vi "RightClickUpdate.vi"(8 "error in (no error)":errorcluster, 10 "Refs":T12, 11 "Loop data in":T1={"TitleCollapse"=refnum, "MouseDownState"=enum."Idle", "RightClickCache"={"Mod"={"Ctrl"=FALSE, "Shift"=FALSE}, "CoordsStart"={"Horizontal"=0, "Vertical"=0}, "CoordsEnd"={"Horizontal"=0, "Vertical"=0}, "PlotAreaBounds"={"Left"=10, "Top"=10, "Right"=0, "Bottom"=0}, "slice"=[]}, "ZoomCache"={"SuppressedPlots"=[], "LeftAxis"={"NeedsRevert?"=FALSE, "Scale Fit"=0, "Range"={"Minimum"=0.0, "Maximum"=0.0, "Increment"=0.0, "Minor Increment"=0.0, "Start"=0.0}}, "RightAxis"={"NeedsRevert?"=FALSE, "Scale Fit"=0, "Range"={"Minimum"=0.0, "Maximum"=0.0, "Increment"=0.0, "Minor Increment"=0.0, "Start"=0.0}}, "Mod"={"Shift"=FALSE}}, "UpdateTime"=0.0, "keyboard"=refnum, "visible?"=FALSE}) -> (0 "error out":errorcluster, 3 "Loop data out":T1={"TitleCollapse"=refnum, "MouseDownState"=enum."Idle", "RightClickCache"={"Mod"={"Ctrl"=FALSE, "Shift"=FALSE}, "CoordsStart"={"Horizontal"=0, "Vertical"=0}, "CoordsEnd"={"Horizontal"=0, "Vertical"=0}, "PlotAreaBounds"={"Left"=10, "Top"=10, "Right"=0, "Bottom"=0}, "slice"=[]}, "ZoomCache"={"SuppressedPlots"=[], "LeftAxis"={"NeedsRevert?"=FALSE, "Scale Fit"=0, "Range"={"Minimum"=0.0, "Maximum"=0.0, "Increment"=0.0, "Minor Increment"=0.0, "Start"=0.0}}, "RightAxis"={"NeedsRevert?"=FALSE, "Scale Fit"=0, "Range"={"Minimum"=0.0, "Maximum"=0.0, "Increment"=0.0, "Minor Increment"=0.0, "Start"=0.0}}, "Mod"={"Shift"=FALSE}}, "UpdateTime"=0.0, "keyboard"=refnum, "visible?"=FALSE})   [LabVIEW 2021, in "RocketPlot.lvlib"]
uses:
  RocketPlot.lvlib
  TypeDefs/Plot UI references.ctl
  Classes/RocketPlotHandle/RocketPlotHandle.lvclass
  <userlib>/bjustice/TipStripOOPanel/Classes/TipPanelHandle/TipPanelHandle.lvclass
  TypeDefs/Plot top row.ctl
  TypeDefs/plot while loop data.ctl
  CollapsePanel/CollapsePanel.lvclass
  TypeDefs/MouseDownState.ctl
  TypeDefs/RightClickCache.ctl
  TypeDefs/RightClickCache PlatMod.ctl
  <vilib>/Utility/miscctls.llb/LVPoint32TypeDef.ctl
  <vilib>/Utility/miscctls.llb/LVRectTypeDef.ctl
  TypeDefs/Slice average.ctl
  TypeDefs/ZoomCache.ctl
  TypeDefs/RangeCache.ctl
  <vilib>/Utility/miscctls.llb/LVRangeTypeDef.ctl
  TypeDefs/ZoomCache PlatMod.ctl
  Plot Load maker V2 - scaleread grid colors.vi
  Classes/TipTablePanel/new cell.vi
  Plot scale refnum to LUT name.vi
  Classes/TipTablePanel/TipTablePanel.lvclass
  C:/Program Files/National Instruments/LabVIEW 2021/user.lib/bjustice/TipStripOOPanel/Classes/TipPanel/TipPanel.lvclass
  <userlib>/bjustice/TipStripOOPanel/Classes/TipPanelHandle/CMD - hide.vi
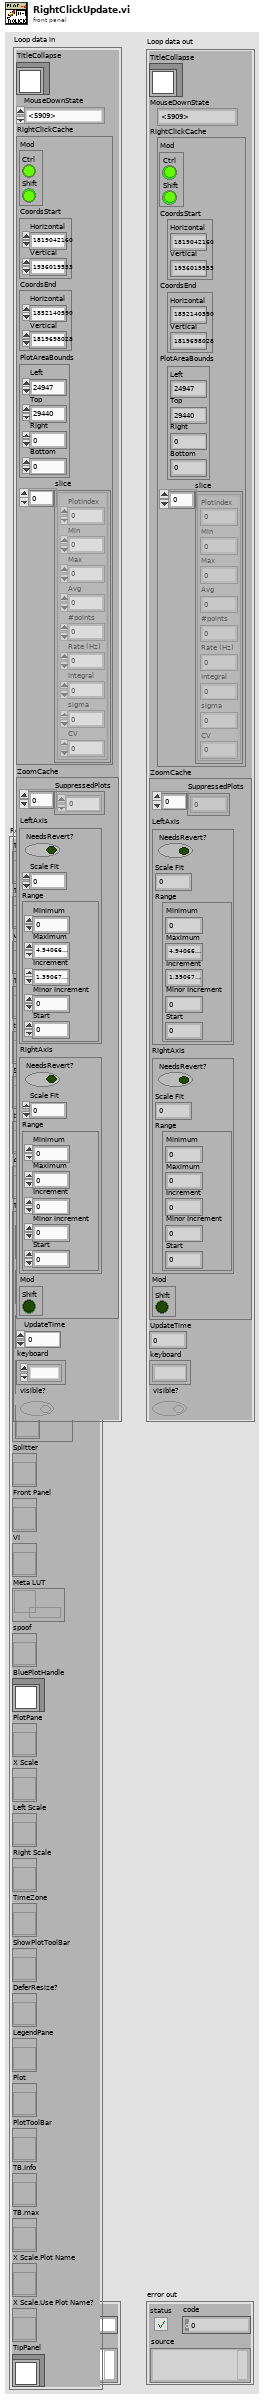
[diagram p1: front panel]
types:
  T1 = typedef "RocketPlot.lvlib/plot while loop data.ctl" = cluster{"TitleCollapse":refnum<class "CollapsePanel.lvclass">, "MouseDownState":T2, "RightClickCache":T3, "ZoomCache":T8, "UpdateTime":dbl, "keyboard":refnum<k1>, "visible?":bool}
  T2 = typedef "RocketPlot.lvlib/MouseDownState.ctl" = enum16{"Idle", "Pan", "Zoom", "Zoom-Post", "RightClick"}
  T3 = typedef "RocketPlot.lvlib/RightClickCache.ctl" = cluster{"Mod":T4, "CoordsStart":T5, "CoordsEnd":T5, "PlotAreaBounds":T6, "slice":T7[]}
  T4 = typedef "RocketPlot.lvlib/RightClickCache PlatMod.ctl" = cluster{"Ctrl":bool, "Shift":bool}
  T5 = typedef "LVPoint32TypeDef.ctl" = cluster{"Horizontal":i32, "Vertical":i32}
  T6 = typedef "LVRectTypeDef.ctl" = cluster{"Left":i16, "Top":i16, "Right":i16, "Bottom":i16}
  T7 = typedef "RocketPlot.lvlib/Slice average.ctl" = cluster{"PlotIndex":i32, "Min":dbl, "Max":dbl, "Avg":dbl, "#points":u32, "Rate (Hz)":dbl, "Integral":dbl, "sigma":dbl, "CV":dbl}
  T8 = typedef "RocketPlot.lvlib/ZoomCache.ctl" = cluster{"SuppressedPlots":i32[], "LeftAxis":T9, "RightAxis":T9, "Mod":T11}
  T9 = typedef "RocketPlot.lvlib/RangeCache.ctl" = cluster{"NeedsRevert?":bool, "Scale Fit":u8, "Range":T10}
  T10 = typedef "LVRangeTypeDef.ctl" = cluster{"Minimum":dbl, "Maximum":dbl, "Increment":dbl, "Minor Increment":dbl, "Start":dbl}
  T11 = typedef "RocketPlot.lvlib/ZoomCache PlatMod.ctl" = cluster{"Shift":bool}
  T12 = typedef "RocketPlot.lvlib/Plot UI references.ctl" = cluster{"Title":refnum<vi>, "Title?":refnum<vi>, "Visible sidebar?":refnum<vi>, "Time to Plot":refnum<vi>, "top array":refnum<vi>, "Scrollbar":refnum<vi>, "tab ref":refnum<vi>, "Add row":refnum<vi>, "TopArray":cluster{"PID":refnum<vi>, "Numeric color":refnum<vi>, "Flat":refnum<vi>, "PID color":refnum<vi>, "Data":refnum<vi>}, "Splitter":refnum<vi>, "Front Panel":refnum<vi>, "VI":refnum<vi>, "Meta LUT":refnum<data-value>, "spoof":refnum<vi>, "BluePlotHandle":refnum<class "RocketPlotHandle.lvclass">, "PlotPane":refnum<vi>, "X Scale":refnum<vi>, "Left Scale":refnum<vi>, "Right Scale":refnum<vi>, "TimeZone":refnum<vi>, "ShowPlotToolBar":refnum<vi>, "DeferResize?":refnum<vi>, "LegendPane":refnum<vi>, "Plot":refnum<vi>, "PlotToolBar":refnum<vi>, "TB.Info":refnum<vi>, "TB.max":refnum<vi>, "X Scale.Plot Name":refnum<vi>, "X Scale.Use Plot Name?":refnum<vi>, "TipPanel":refnum<class "TipPanelHandle.lvclass">}
  T13 = typedef "RocketPlot.lvlib/RightClickType.ctl" = enum16{"Idle", "Delta", "SliceAvg", "Identify"}
  T14 = typedef "RocketPlot.lvlib/TipTablePanel.lvclass/cell cache.ctl" = cluster{"text":string, "Color":u32, "Justification":enum16{"Left", "Center", "Right"}}
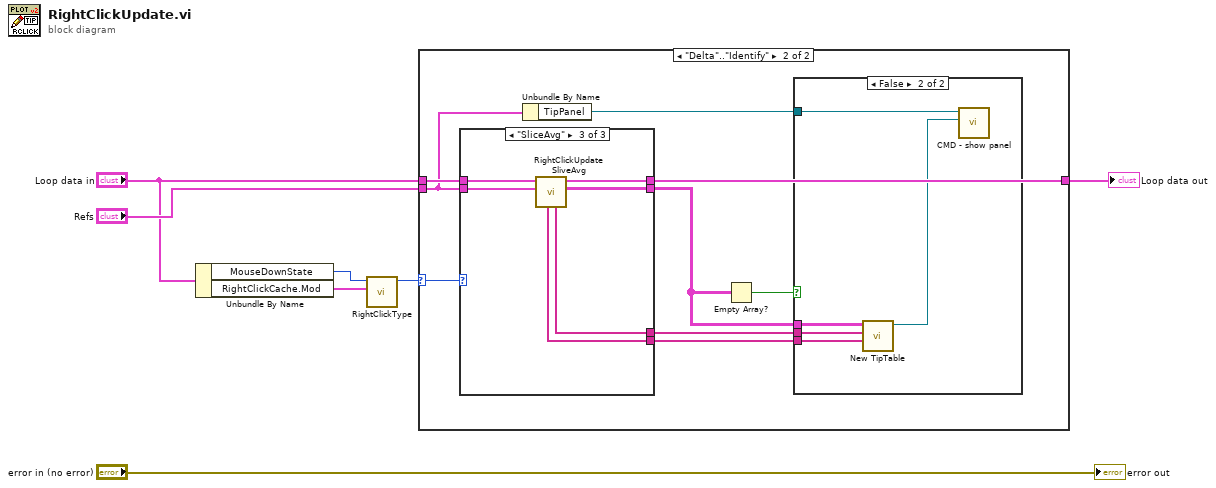
[diagram p0: block diagram]
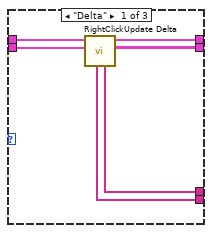
[diagram p3: hidden frame]
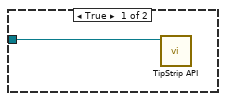
[diagram p5: hidden frame]
diagram:
  n1 = Unbundle By Name("Loop data in") -> ("MouseDownState"=w4:T2, "RightClickCache.Mod"=w5:T4)
  n2 = call "RightClickType.vi"("Mod"=w5, "MouseDownState"=w4) -> ("RightClickType"=w3:T13)  [unwired: 9 in]
  n3 = case shown="\"Delta\"..\"Identify\"" w3 {
    selector: w3 -> [_ w11]
    tunnel: "Refs" -> [_ w10]
    tunnel: "Loop data in" -> [w8 w16]
    tunnel: [w8 w12] -> w1
    frame "Idle" {
    }
    frame "Delta".."Identify" {
      n4 = case shown="\"SliceAvg\"" w11 {
        tunnel: w16 -> [w23 w24 w30]
        tunnel: w10 -> [w22 _ w28]
        tunnel: [w21 _ w27] -> w15
        tunnel: [w20 _ w25] -> w14
        tunnel: [w19 _ w26] -> w13
        tunnel: [w18 w24 w29] -> w12
        frame "Delta" {
          n5 = call "RightClickUpdate Delta.vi"("Refs"=w22, "Loop data in"=w23) -> ("cells"=w21:T14[][], "Loop data out"=w18:T1, "Row Headers"=w20:string[], "Column Headers"=w19:string[])  [unwired: 5 in, 1 out]
        }
        frame Default {
        }
        frame "SliceAvg" {
          n6 = call "RightClickUpdate SliveAvg.vi"("Refs"=w28, "Loop data in"=w30) -> ("cells"=w27:T14[][], "Loop data out"=w29:T1, "Row Headers"=w25:string[], "Column Headers"=w26:string[])  [unwired: 5 in, 1 out]
        }
      }
      n7 = Unbundle By Name(w10) -> ("TipPanel"=w9:refnum<class "TipPanelHandle.lvclass">)
      n8 = Empty Array?(array=w15) -> (empty?=w17:bool)
      n9 = case shown="False" w17 {
        tunnel: w14 -> [_ w35]
        tunnel: w13 -> [_ w34]
        tunnel: w15 -> [_ w36]
        tunnel: w9 -> [w31 w33]
        frame True {
          n10 = call-poly <userlib>:"TipStrip API.vi"("TipPanelHandle"=w31) -> ()  [unwired: 9 in, 2 out]
        }
        frame False {
          n11 = call "New TipTable.vi"("show.Column Headers"=w34, "show.Row Headers"=w35, "show.cells"=w36) -> ("TipTablePanel out"=w32:refnum<class "TipTablePanel.lvclass">)  [unwired: 7 in, 1 out]
          n12 = call <userlib>:"CMD - show panel.vi"("TipPanel"=w32, "TipPanelHandle"=w33) -> ()  [unwired: 8 in, 2 out]
        }
      }
    }
  }
  "Loop data out" <- w1
  "error out" <- "error in (no error)"
